vi "LVClass_HasoSlopes Read HasoSlopes _ property.vi"(8 "error in (no error)":errorcluster, 11 "HasoSlopes in":refnum<class "HasoSlopes.lvclass">) -> (0 "error out":errorcluster, 2 "ClassID_void":T1, 3 "HasoSlopes out":refnum<class "HasoSlopes.lvclass">)   [LabVIEW 2020, in "HasoSlopes.lvclass"]
uses:
  HasoSlopes.lvclass
  ClassID.ctl
  HasoSlopes.lvclass/HasoSlopes.ctl
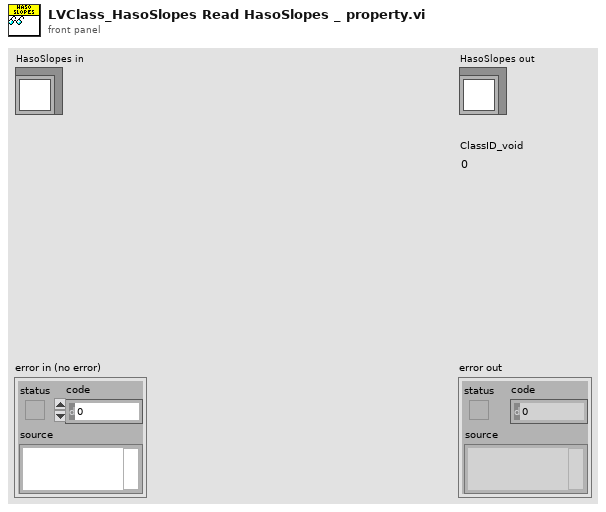
[diagram p1: front panel]
types:
  T1 = typedef "ClassID.ctl" = i64
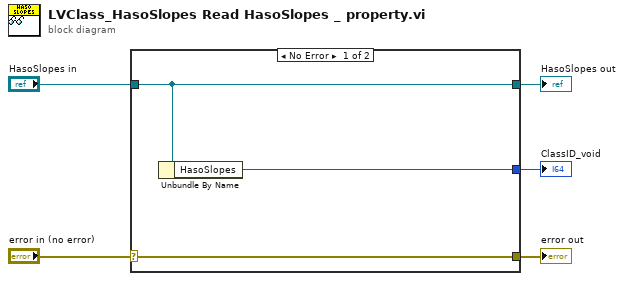
[diagram p0: block diagram]
diagram:
  n1 = case shown="No Error" "error in (no error)" {
    selector: "error in (no error)" -> [w8 w9]
    tunnel: [w8 w9] -> w4
    tunnel: [w7 w10] -> w2
    tunnel: "HasoSlopes in" -> [w7 w10]
    tunnel: [w6 _] -> w1
    frame No Error {
      n2 = Unbundle By Name(w7) -> ("HasoSlopes"=w6:T1)
    }
    frame Error {
    }
  }
  "error out" <- w4
  "HasoSlopes out" <- w2
  "ClassID_void" <- w1
